vi "console.vi"() -> ()   [LabVIEW 2021]
panel:
  out "Console":string
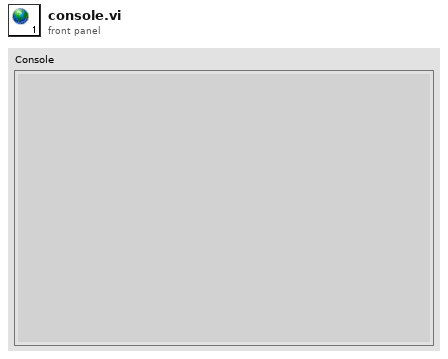
[diagram p1: front panel]
diagram:
